vi "FP_Watcher.vi"(9 "W_out":dbl, 10 "V_out":dbl, 11 "Current_Position_out":T1) -> (3 "Watcher":T2)   [LabVIEW 2017]
uses:
  Ctl/Current_Position.ctl
  GBL/GBL_variables.vi
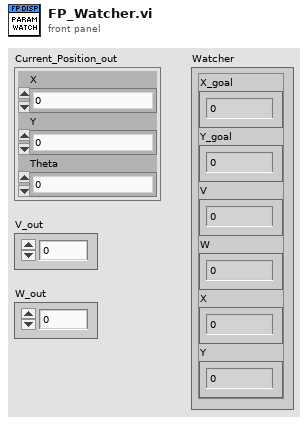
[diagram p1: front panel]
types:
  T1 = typedef "Current_Position.ctl" = cluster{"X":dbl, "Y":dbl, "Theta":dbl}
  T2 = cluster{"X_goal":dbl, "Y_goal":dbl, "V":dbl, "W":dbl, "X":dbl, "Y":dbl}
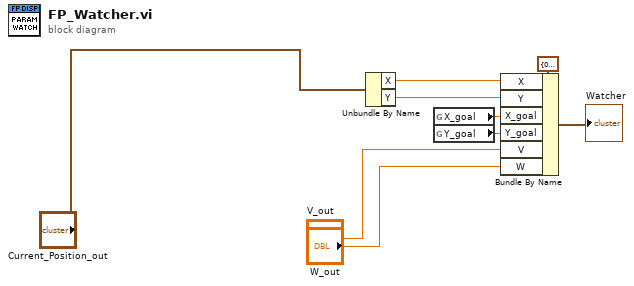
[diagram p0: block diagram]
diagram:
  n1 = Unbundle By Name("Current_Position_out") -> ("X"=w7:dbl, "Y"=w8:dbl)
  n2 = global read "GBL_variables.vi" "X_goal"() -> (w2:dbl)
  n3 = global read "GBL_variables.vi" "Y_goal"() -> (w1:dbl)
  n4 = Bundle By Name(cluster=T2 {"X_goal"=0.0, "Y_goal"=0.0, "V"=0.0, "W"=0.0, "X"=0.0, "Y"=0.0} ("Watcher"), "X"=w7, "Y"=w8, "X_goal"=w2, "Y_goal"=w1, "V"="V_out", "W"="W_out") -> (→"Watcher":T2)
